vi "Decompress.vi"(8 "error in (no error)":errorcluster, 11 "compressed data":u8[](array[numeric])) -> (0 "error out":errorcluster, 3 "data":u8[](array[numeric]))   [LabVIEW 2020, in "GZip.lvclass"]
uses:
  GZip.lvclass
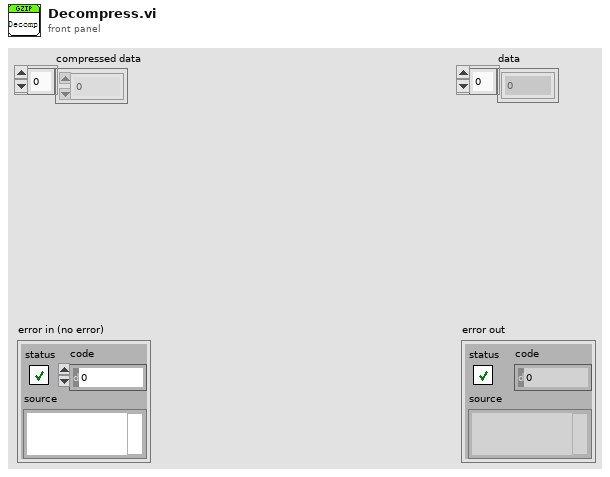
[diagram p1: front panel]
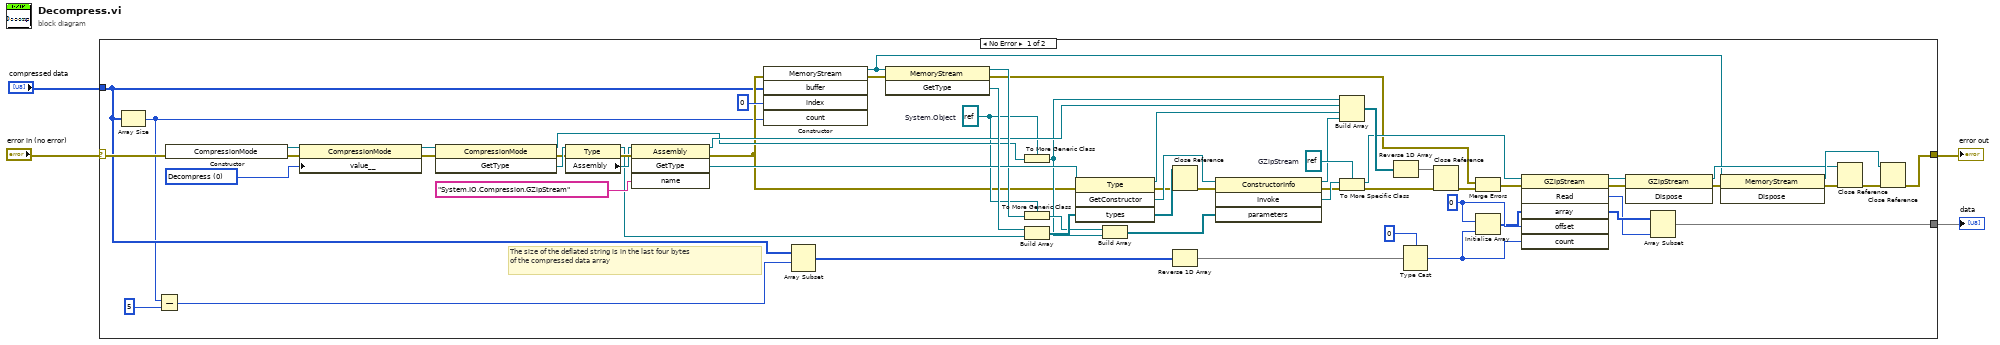
[diagram p0: block diagram]
diagram:
  n1 = case shown="No Error" "error in (no error)" {
    selector: "error in (no error)" -> [w8 w68]
    tunnel: [w52 w68] -> w2
    tunnel: "compressed data" -> [w7 _]
    tunnel: [w5 _] -> w1
    frame No Error {
      w17 = 0 items=["Decompress", "Compress"] ("CompressionMode in")
      w10 = refnum<k24> refnum  # System.Object
      w32 = refnum<k24> refnum  # GZipStream
      w56 = u8 0 ("offset")
      # "The size of the deflated string is in the last four bytes \nof the compressed data array"
      n2 = Array Size(array=w7) -> (size(s)=w6:i32)
      n3 = Subtract(x=w6, y=5) -> (x-y=w63:i32)
      n4 = constructor class="CompressionMode"(error in=w8) -> (reference out=w36:refnum<k24>, error out=w43:errorcluster)  [unwired: 2 in, 1 out]
      n5 = property class="CompressionMode"(reference=w36, error in=w43, "value__"=w17) -> (reference out=w35:refnum<k24>, error out=w37:errorcluster)
      n6 = invoke class="CompressionMode" method="GetType"(reference=w35, error in=w37) -> (reference out=w19:refnum<k24>, error out=w41:errorcluster, "GetType"=w42:refnum<k24>)  [unwired: 1 in]
      n7 = property class="Type"(reference=w42, error in=w41) -> (reference out=w38:refnum<k24>, error out=w40:errorcluster, "Assembly"=w39:refnum<k24>)
      n8 = invoke class="Assembly" method="GetType"(reference=w39, error in=w40, "name"="System.IO.Compression.GZipStream") -> (reference out=w20:refnum<k24>, error out=w9:errorcluster, "GetType"=w45:refnum<k24>)  [unwired: 1 in, 1 out]
      n9 = constructor class="MemoryStream"(error in=w9, "buffer"=w7, "index"=0, "count"=w6) -> (reference out=w16:refnum<k24>, error out=w15:errorcluster)  [unwired: 2 in, 4 out]
      n10 = Array Subset(array=w7, index=w63) -> (w64:u8[])  [unwired: 1 in]
      n11 = invoke class="MemoryStream" method="GetType"(reference=w16, error in=w15) -> (reference out=w25:refnum<k24>, error out=w11:errorcluster, "GetType"=w47:refnum<k24>)  [unwired: 1 in]
      n12 = To More Generic Class(target class=w10, reference=w19) -> (generic class reference=w18:refnum<k24>)
      n13 = To More Generic Class(target class=w10, reference=w25) -> (generic class reference=w24:refnum<k24>)
      n14 = Build Array(w47, w38) -> (w46:refnum<k24>[])
      n15 = invoke class="Type" method="GetConstructor"(reference=w45, error in=w9, "types"=w46) -> (reference out=w21:refnum<k24>, error out=w28:errorcluster, "GetConstructor"=w44:refnum<k24>, "types"=w29:refnum<k24>[])  [unwired: 1 in]
      n16 = Build Array(w24, w18) -> (w34:refnum<k24>[])
      n17 = Close Reference(reference=w29, error in (no error)=w28) -> (error out=w27:errorcluster)
      n18 = Reverse 1D Array(array=w64) -> (reversed array=w65:u8[])
      n19 = invoke class="ConstructorInfo" method="Invoke"(reference=w44, error in=w27, "parameters"=w34) -> (reference out=w22:refnum<k24>, error out=w31:errorcluster, "Invoke"=w33:refnum<k24>)  [unwired: 1 in, 1 out]
      n20 = Build Array(w18, w20, w21, w22) -> (w30:refnum<k24>[])
      n21 = To More Specific Class(target class=w32, reference=w33, error in=w31) -> (specific class reference=w14:refnum<k24>, error out=w26:errorcluster)
      n22 = Reverse 1D Array(array=w30) -> (reversed array=w23:refnum<k24>[])
      n23 = Type Cast(type=u32 0, x=w65) -> (*(type *) &x=w67:u32)
      n24 = Close Reference(reference=w23, error in (no error)=w26) -> (error out=w13:errorcluster)
      n25 = Merge Errors(w11, w13) -> (w12:errorcluster)
      n26 = Initialize Array(w56, w67) -> (w55:u8[])
      n27 = invoke class="GZipStream" method="Read"(reference=w14, error in=w12, "array"=w55, "offset"=w56, "count"=w67) -> (reference out=w58:refnum<k24>, error out=w59:errorcluster, "Read"=w54:i32, "array"=w57:u8[])  [unwired: 1 in, 2 out]
      n28 = invoke class="GZipStream" method="Dispose"(reference=w58, error in=w59) -> (reference out=w49:refnum<k24>, error out=w60:errorcluster)  [unwired: 1 in, 1 out]
      n29 = Array Subset(array=w57, length=w54) -> (w5:u8[])  [unwired: 1 in]
      n30 = invoke class="MemoryStream" method="Dispose"(reference=w16, error in=w60) -> (reference out=w53:refnum<k24>, error out=w51:errorcluster)  [unwired: 1 in, 1 out]
      n31 = Close Reference(reference=w49, error in (no error)=w51) -> (error out=w50:errorcluster)
      n32 = Close Reference(reference=w53, error in (no error)=w50) -> (error out=w52:errorcluster)
    }
    frame Error {
    }
  }
  "error out" <- w2
  "data" <- w1
